vi "Get cif_launcher_DiscoveredPlugin.vi"(8 "error in (no error)":errorcluster, 11 "gRPCid":T1) -> (0 "error out":errorcluster, 2 "package_templatemessage":T2, 3 "gRPCid out":T1)   [LabVIEW 2021, in "CIF_Launcher_server.lvlib"]
uses:
  CIF_Launcher_server.lvlib
  cif_launcher_DiscoveredPlugin.ctl
  cif_common_Version.ctl
  cif_manager_PluginMetadata.ctl
  <vilib>/gRPC/LabVIEW gRPC Library/Shared/grpcId.ctl
  cif_launcher_DiscoveredPlugin_Flat.ctl
  cif_common_Version_Flat.ctl
  cif_manager_PluginMetadata_Flat.ctl
  2ed25e12-861d-4677-8ead-ace2906b2041.vi
  <vilib>/gRPC/LabVIEW gRPC Library/Shared/TranslateGrpcError.vi
  FlatToRichcif_common_Version.vi
  FlatToRichcif_manager_PluginMetadata.vi
  <vilib>/gRPC/LabVIEW gRPC Library/Server API/Server/Get Server DLL Path.vi
  <vilib>/Utility/error.llb/Error Cluster From Error Code.vi
  <vilib>/gRPC/LabVIEW gRPC Library/grpc-lvsupport-release.lvlib
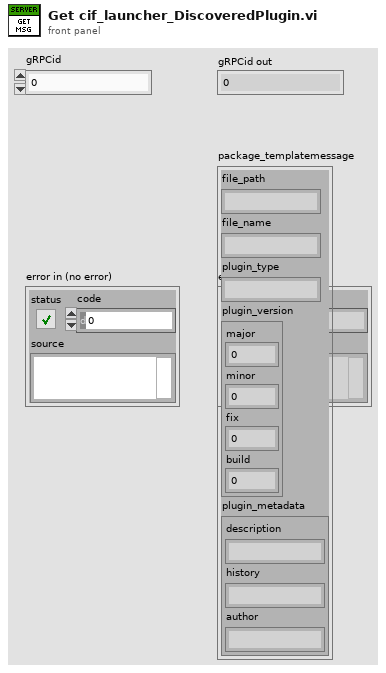
[diagram p1: front panel]
types:
  T1 = typedef "grpc-lvsupport-release.lvlib/grpcId.ctl" = u64
  T2 = typedef "CIF_Launcher_server.lvlib/cif_launcher_DiscoveredPlugin.ctl" = cluster{"file_path":string, "file_name":string, "plugin_type":string, "plugin_version":T3, "plugin_metadata":T4}
  T3 = typedef "CIF_Launcher_server.lvlib/cif_common_Version.ctl" = cluster{"major":u32, "minor":u32, "fix":u32, "build":u32}
  T4 = typedef "CIF_Launcher_server.lvlib/cif_manager_PluginMetadata.ctl" = cluster{"description":string, "history":string, "author":string}
  T5 = typedef "CIF_Launcher_server.lvlib/cif_launcher_DiscoveredPlugin_Flat.ctl" = cluster{"file_path":string, "file_name":string, "plugin_type":string, "plugin_version":T6, "plugin_metadata":T7}
  T6 = typedef "CIF_Launcher_server.lvlib/cif_common_Version_Flat.ctl" = cluster{"major":u32, "minor":u32, "fix":u32, "build":u32}
  T7 = typedef "CIF_Launcher_server.lvlib/cif_manager_PluginMetadata_Flat.ctl" = cluster{"description":string, "history":string, "author":string}
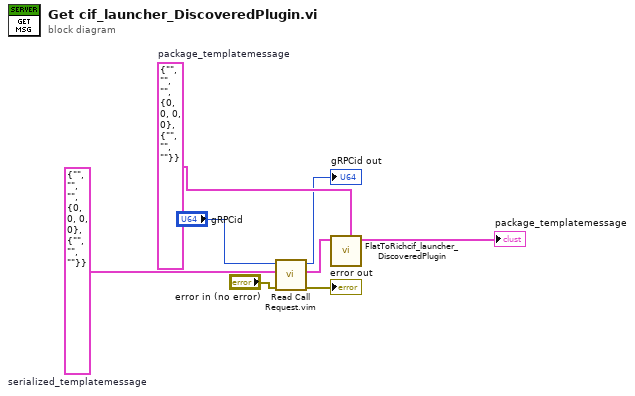
[diagram p0: block diagram]
diagram:
  w6 = T5 {"file_path"="", "file_name"="", "plugin_type"="", "plugin_version"={"major"=0, "minor"=0, "fix"=0, "build"=0}, "plugin_metadata"={"description"="", "history"="", "author"=""}}  # serialized_templatemessage
  w5 = T2 {"file_path"="", "file_name"="", "plugin_type"="", "plugin_version"={"major"=0, "minor"=0, "fix"=0, "build"=0}, "plugin_metadata"={"description"="", "history"="", "author"=""}}  # package_templatemessage
  n1 = call "Read Call Request.vim"("error in"="error in (no error)", "Request Type"=w6, "gRPCid in"="gRPCid") -> ("error out"=→"error out":errorcluster, "Request Data"=w4:T5, "gRPCid out"=→"gRPCid out":T1)  [unwired: 6 in]
  n2 = call "FlatToRichcif_launcher_DiscoveredPlugin.vi"("OutputClusterType"=w5, "InputCluster"=w4) -> ("OutputCluster"=→"package_templatemessage":T2)  [unwired: 9 in]
